vi "subsystem_Connect.vi"(8 "error in (no":errorcluster, 11 "ProgrammaticInitialization in":refnum<class "ProgrammaticInitialization.lvclass">) -> (0 "error out":errorcluster, 3 "ProgrammaticInitialization out":refnum<class "ProgrammaticInitialization.lvclass">)   [LabVIEW 2016, in "ProgrammaticInitialization.lvclass"]
uses:
  ProgrammaticInitialization.lvclass
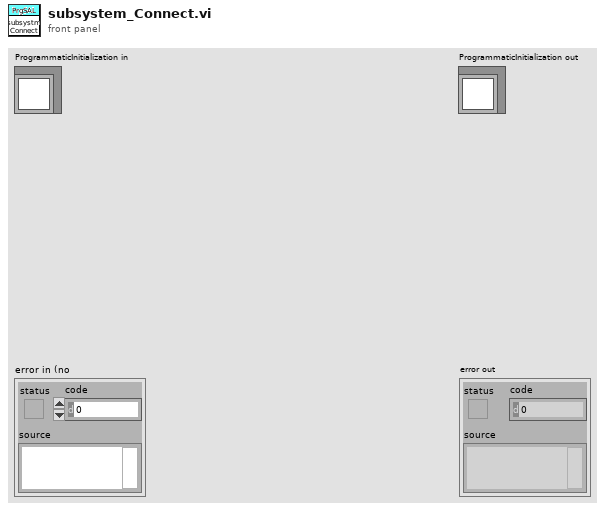
[diagram p1: front panel]
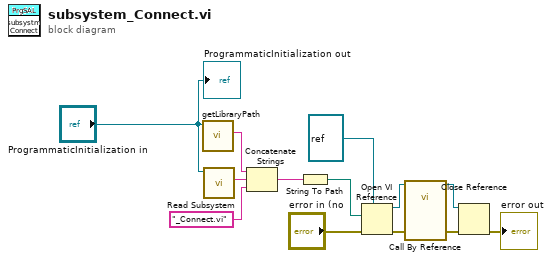
[diagram p0: block diagram]
diagram:
  n1 = call "getLibraryPath.vi"("ProgrammaticInitialization in"="ProgrammaticInitialization in") -> ("SAL_Library"=w3:string)  [unwired: 8 in, 2 out]
  n2 = call-dynamic "Read Subsystem.vi"("ProgrammaticInitialization in"="ProgrammaticInitialization in") -> ("Subsystem"=w6:string)  [unwired: 8 in, 2 out]
  n3 = Concatenate Strings(w3, w6, "_Connect.vi" ("string")) -> (w1:string)
  n4 = String To Path(string=w1) -> (path=w2:path)
  n5 = Open VI Reference(type specifier VI Refnum (for type only)=refnum<vi> refnum, vi path=w2, error in (no error)="error in (no") -> (vi reference=w13:refnum<vi>, error out=w8:errorcluster)  [unwired: 3 in]
  n6 = call-by-ref "?"(reference=w13, "error in (no error)"=w8) -> (reference out=w12:refnum<vi>, "error out"=w7:errorcluster)  [unwired: 10 in, 2 out]
  n7 = Close Reference(reference=w12, error in (no error)=w7) -> (error out=→"error out":errorcluster)
  "ProgrammaticInitialization out" <- "ProgrammaticInitialization in"
